vi "Error Handler.vi"(8 "Engine Error":errorcluster, 11 "Component Info In":T1) -> (0 "Engine Errors":errorcluster, 1 "Safe State":bool, 3 "Component Info Out":T1)   [LabVIEW 2013]
uses:
  Module Execution Info.ctl
  <vilib>/NI/Tag Bus Module Framework/runtime/TBM module execution interface.lvclass
  Data Table with Transfer Spec.ctl
  <vilib>/NI/Tag Bus/table/data table.ctl
  <vilib>/NI/Tag Bus/table/transfer specification.ctl
  <vilib>/NI/Tag Bus/tag/Data Type.ctl
  Configuration/Module Decimation.ctl
  Configuration/Module Error Configuration.ctl
  Configuration/Error Actions By Category.ctl
  <vilib>/NI/Tag Bus Module Framework/runtime/error classification.ctl
  Configuration/Error Actions.ctl
  error responses.ctl
  Configuration/error options.ctl
  Standard Engine Runtime.lvclass
  Configuration/Standard Engine Configuration.lvclass
  <vilib>/NI/Tag Bus/tag/tag descriptor.lvclass
  <vilib>/NI/Tag Bus/table/data table.lvlib
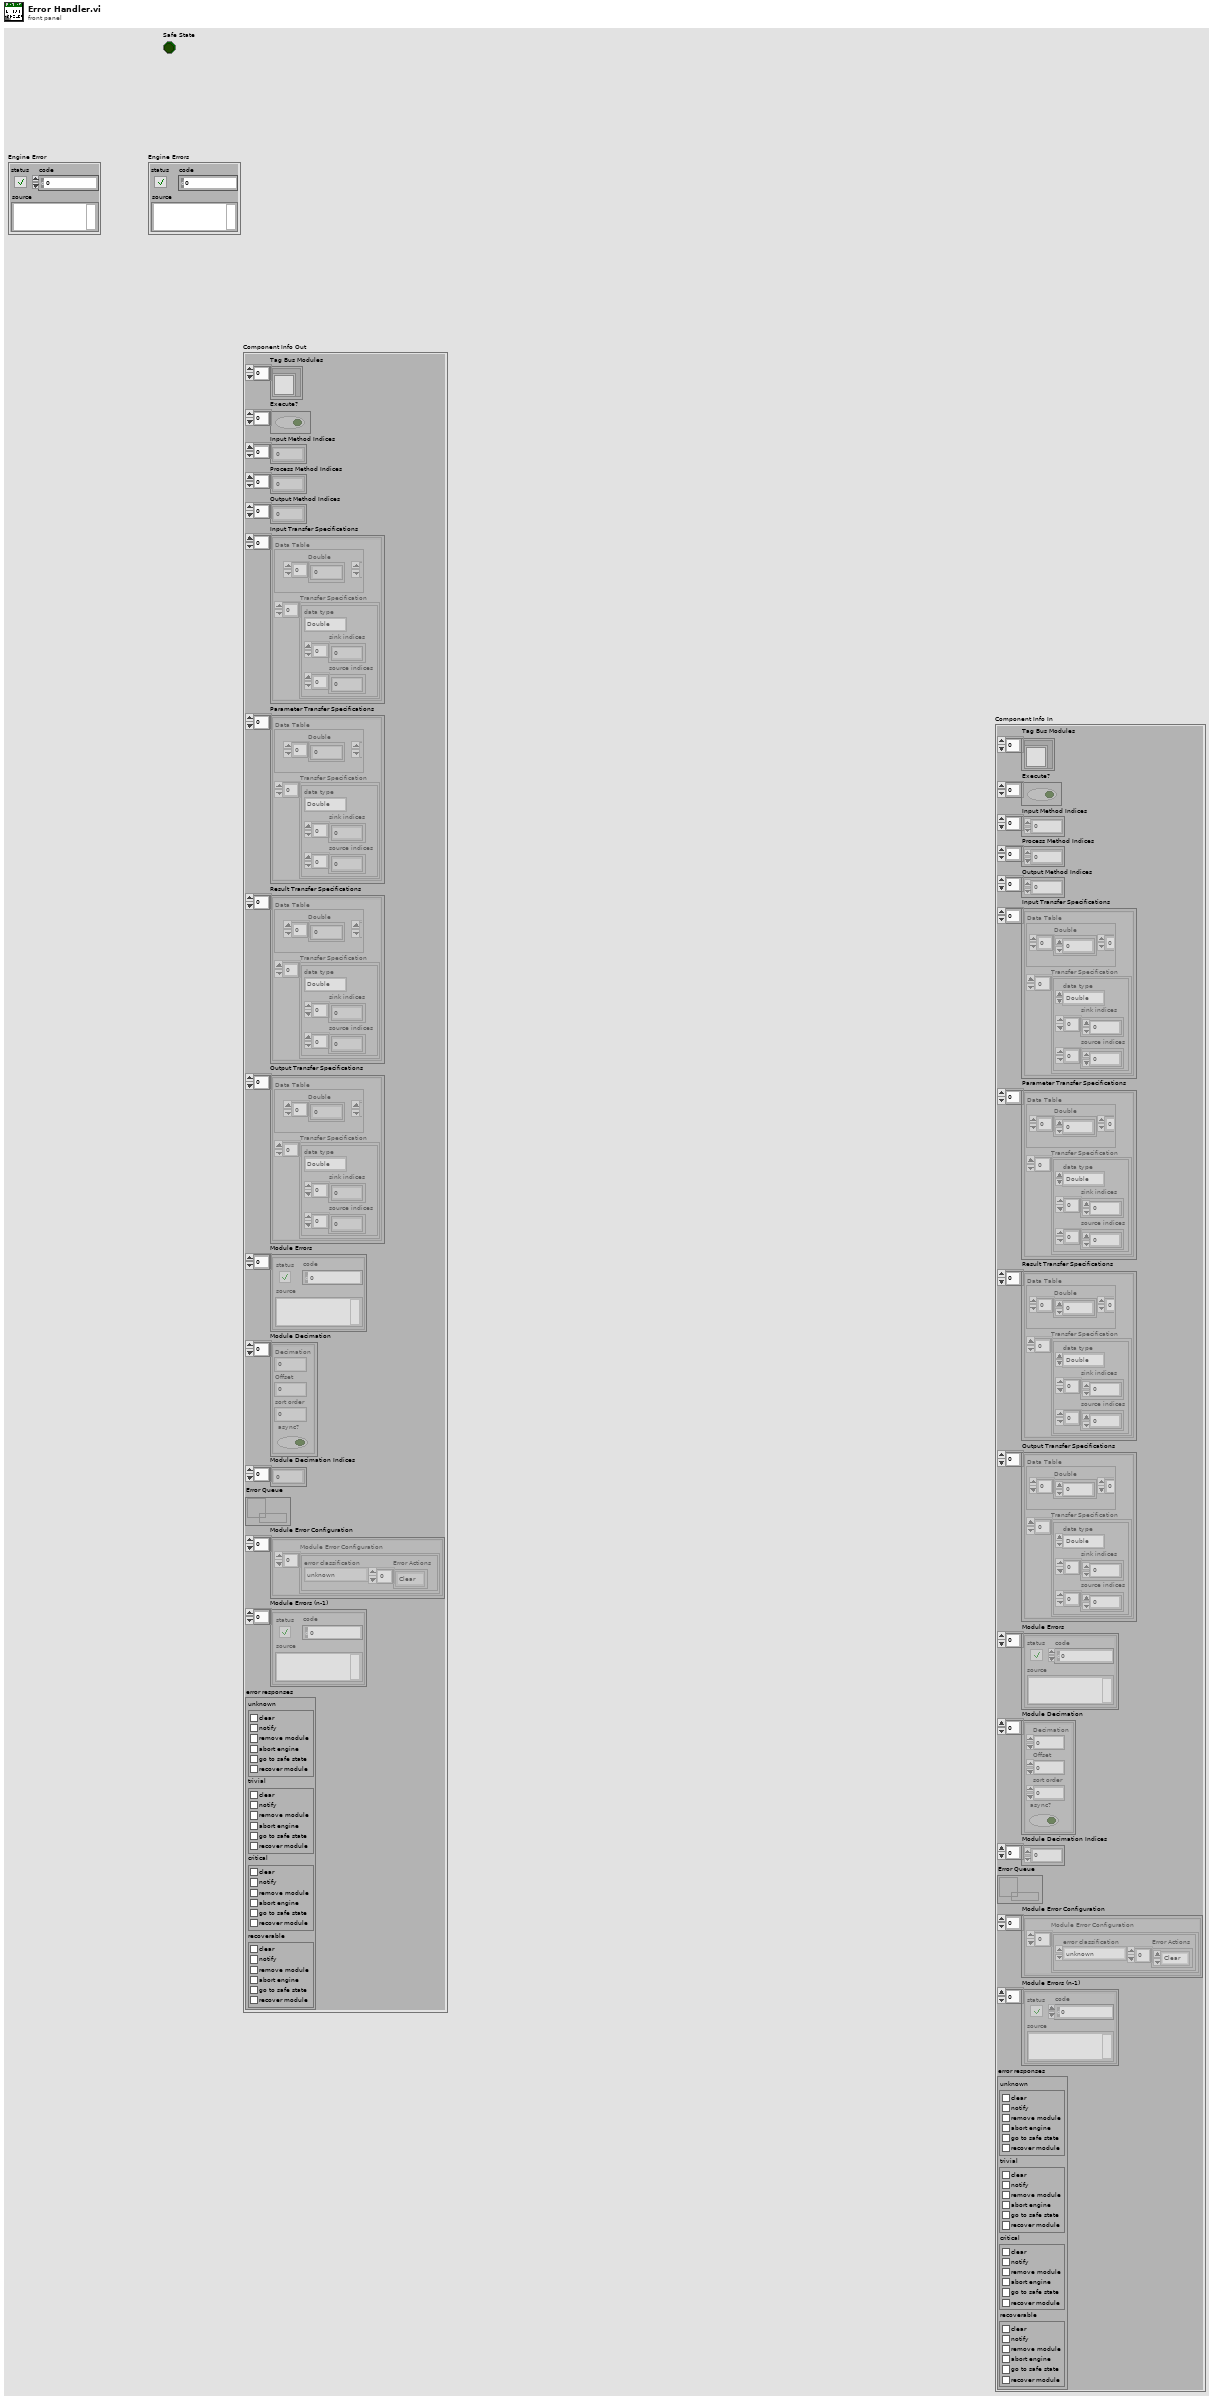
[diagram p1: front panel]
types:
  T1 = typedef "Module Execution Info.ctl" = cluster{"Tag Bus Modules":refnum<class "TBM module execution interface.lvclass">[], "Execute?":bool[], "Input Method Indices":i32[], "Process Method Indices":i32[], "Output Method Indices":i32[], "Input Transfer Specifications":T2[], "Parameter Transfer Specifications":T2[], "Result Transfer Specifications":T2[], "Output Transfer Specifications":T2[], "Module Errors":errorcluster[], "Module Decimation":T6[], "Module Decimation Indices":i32[], "Error Queue":refnum<queue>, "Module Error Configuration":T7[], "Module Errors (n-1)":errorcluster[], "error responses":T11}
  T2 = typedef "Data Table with Transfer Spec.ctl" = cluster{"Data Table":T3, "Transfer Specification":T4[]}
  T3 = typedef "tag bus.lvlib/data table.lvlib/data table.ctl" = cluster{"Double":dbl[], "Single":sgl[], "I64":i64[], "I32":i32[], "I16":i16[], "I8":i8[], "U64":u64[], "U32":u32[], "U16":u16[], "U8":u8[], "Boolean":bool[], "String":string[], "Array of Double":cluster{"DBL Array":dbl[]}[], "Array of Single":cluster{"SGL Array":sgl[]}[], "Array of I64":cluster{"I64 Array":i64[]}[], "Array of I32":cluster{"I32 Array":i32[]}[], "Array of I16":cluster{"I16 Array":i16[]}[], "Array of I8":cluster{"I8 Array":i8[]}[], "Array of U64":cluster{"U64 Array":u64[]}[], "Array of U32":cluster{"U32 Array":u32[]}[], "Array of U16":cluster{"U16 Array":u16[]}[], "Array of U8":cluster{"U8 Array":u8[]}[], "Array of Boolean":cluster{"Boolean Array":bool[]}[], "Array of String":cluster{"String Array":string[]}[]}
  T4 = typedef "tag bus.lvlib/data table.lvlib/transfer specification.ctl" = cluster{"data type":T5, "sink indices":i32[], "source indices":i32[]}
  T5 = typedef "tag bus.lvlib/tag descriptor.lvclass/Data Type.ctl" = enum16{"Double", "Single", "I64", "I32", "I16", "I8", "U64", "U32", "U16", "U8", "Boolean", "String", "Array of Double", "Array of Single", "Array of I64", "Array of I32", "Array of I16", "Array of I8", "Array of U64", "Array of U32", "Array of U16", "Array of U8", "Array of Boolean", "Array of String"}
  T6 = typedef "Standard Engine Configuration.lvclass/Module Decimation.ctl" = cluster{"Decimation":u16, "Offset":u16, "sort order":i32, "async?":bool}
  T7 = typedef "Standard Engine Configuration.lvclass/Module Error Configuration.ctl" = cluster{"Module Error Configuration":T8[]}
  T8 = typedef "Standard Engine Configuration.lvclass/Error Actions By Category.ctl" = cluster{"error classification":T9, "Error Actions":T10[]}
  T9 = typedef "TBM module execution interface.lvclass/error classification.ctl" = enum16{"unknown", "none", "trivial", "recoverable", "critical"}
  T10 = typedef "Standard Engine Configuration.lvclass/Error Actions.ctl" = enum16{"Clear", "Notify", "Stop Component", "Stop Engine", "Safe State", "Attempt Recovery"}
  T11 = typedef "Standard Engine Configuration.lvclass/error responses.ctl" = cluster{"unknown":T12, "trivial":T12, "critical":T12, "recoverable":T12}
  T12 = typedef "Standard Engine Configuration.lvclass/error options.ctl" = cluster{"clear":bool, "notify":bool, "remove module":bool, "abort engine":bool, "go to safe state":bool, "recover module":bool}
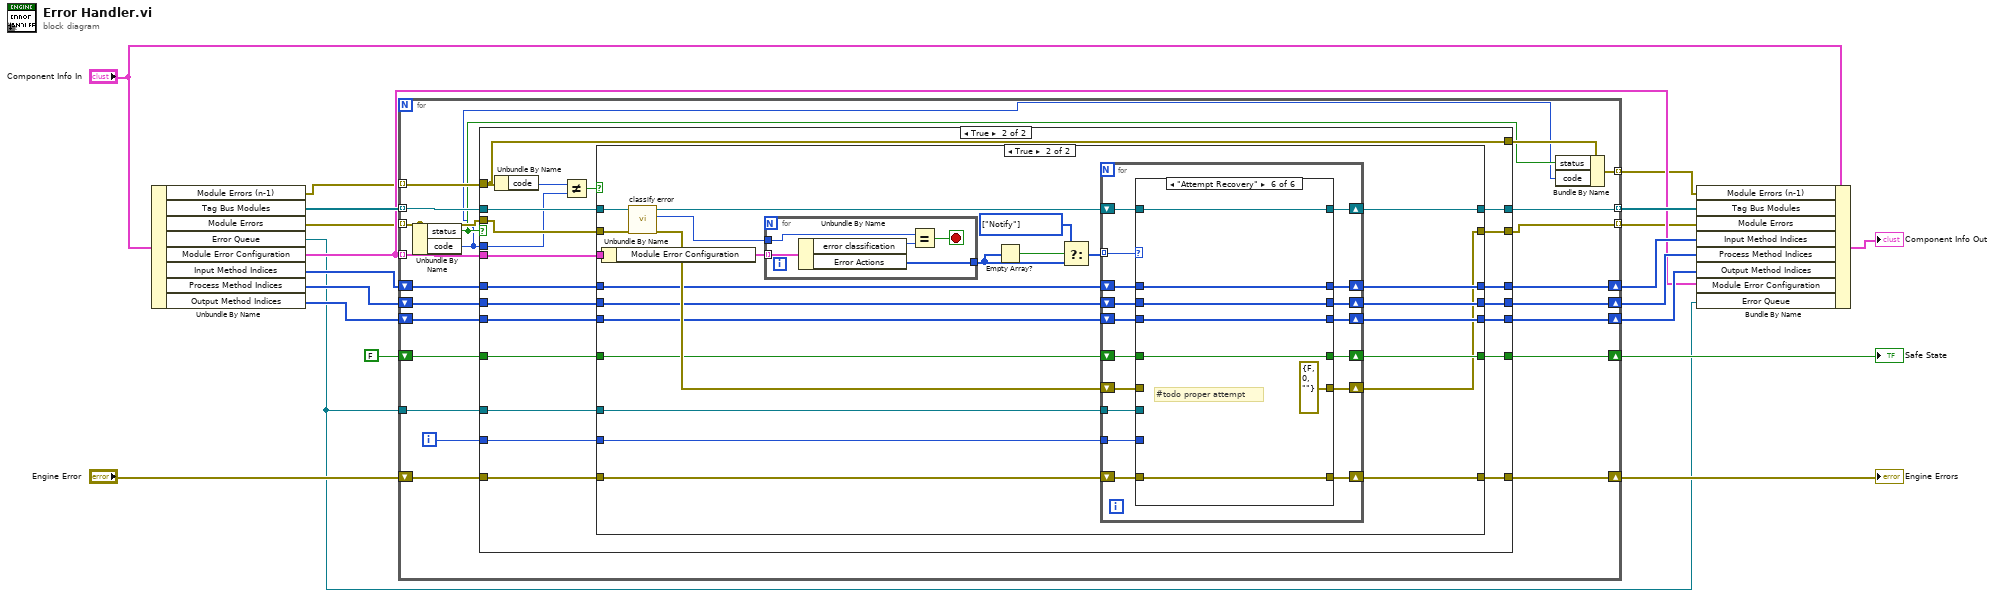
[diagram p0: block diagram]
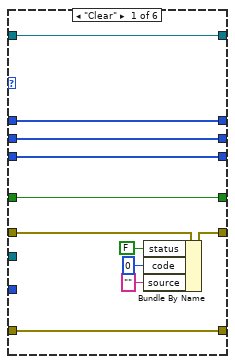
[diagram p4: hidden frame]
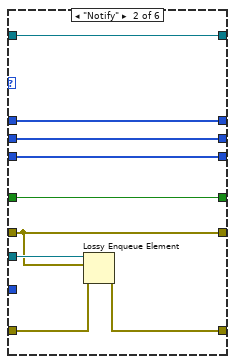
[diagram p5: hidden frame]
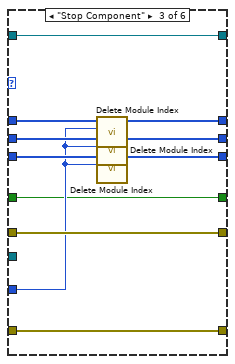
[diagram p6: hidden frame]
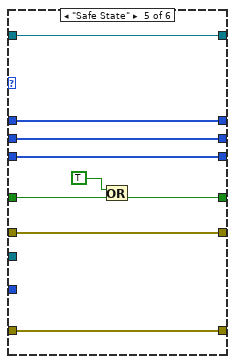
[diagram p8: hidden frame]
diagram:
  n1 = Unbundle By Name("Component Info In") -> ("Module Errors (n-1)"=w3:errorcluster[], "Tag Bus Modules"=w18:refnum<class "TBM module execution interface.lvclass">[], "Module Errors"=w4:errorcluster[], "Error Queue"=w5:refnum<queue>, "Module Error Configuration"=w6:T7[], "Input Method Indices"=w14:i32[], "Process Method Indices"=w13:i32[], "Output Method Indices"=w12:i32[])
  n2 = for {
    tunnel: w4 -> [w24] mode=indexing
    tunnel: [w40] -> w16 mode=indexing
    tunnel: w18 -> [w38] mode=indexing
    tunnel: w6 -> [w39] mode=indexing
    shift-right: [w41] -> w20
    shift-left: "Engine Error" -> [w42]
    tunnel: w5 -> [w37]
    shift-right: [w33] -> w11
    shift-left: w14 -> [w36]
    shift-right: [w32] -> w10
    shift-left: w13 -> [w35]
    shift-right: [w31] -> w9
    shift-left: w12 -> [w34]
    tunnel: w3 -> [w30] mode=indexing
    shift-right: [w29] -> w7
    shift-left: FALSE -> [w28]
    tunnel: [w26] -> w2 mode=indexing
    tunnel: [w23] -> w1 mode=indexing
    i -> [w25]
    n3 = Unbundle By Name(w24) -> ("status"=w22:bool, "code"=w21:i32)
    n4 = case shown="True" w22 {
      tunnel: w42 -> [w50 w68]
      tunnel: [w50 w67] -> w41
      tunnel: [w43 w70] -> w26
      tunnel: [w49 w69] -> w40
      tunnel: w38 -> [w49 w71]
      tunnel: w39 -> [_ w58]
      tunnel: w37 -> [_ w66]
      tunnel: w36 -> [w48 w65]
      tunnel: w35 -> [w47 w64]
      tunnel: w34 -> [w46 w63]
      tunnel: [w48 w62] -> w33
      tunnel: [w47 w61] -> w32
      tunnel: [w46 w60] -> w31
      tunnel: w25 -> [_ w59]
      tunnel: w30 -> [w44 w53]
      tunnel: [w45 w54] -> w29
      tunnel: w28 -> [w45 w55]
      tunnel: [w44 w53] -> w27
      tunnel: w24 -> [w43 w52]
      tunnel: w21 -> [_ w51]
      frame False {
      }
      frame True {
        n5 = Unbundle By Name(w53) -> ("code"=w57:i32)
        n6 = Not Equal?(x=w57, y=w51) -> (x != y?=w56:bool)
        n7 = case shown="True" w56 {
          tunnel: w71 -> [w78 w103]
          tunnel: [w77 w79] -> w70
          tunnel: [w78 w100] -> w69
          tunnel: w68 -> [w73 w99]
          tunnel: [w73 w98] -> w67
          tunnel: w66 -> [_ w97]
          tunnel: w65 -> [w76 w96]
          tunnel: w64 -> [w75 w95]
          tunnel: w63 -> [w74 w94]
          tunnel: [w76 w93] -> w62
          tunnel: [w75 w92] -> w61
          tunnel: [w74 w91] -> w60
          tunnel: w59 -> [_ w90]
          tunnel: w58 -> [_ w89]
          tunnel: w52 -> [w77 w82]
          tunnel: w55 -> [w72 w81]
          tunnel: [w72 w80] -> w54
          frame False {
          }
          frame True {
            w83 = T10[] [enum."Notify"] items=["Clear", "Notify", "Stop Component", "Stop Engine", "Safe State", "Attempt Recovery"] ("t")
            n8 = Unbundle By Name(w89) -> ("Module Error Configuration"=w88:T8[])
            n9 = call-dynamic "classify error.vi"("error to classify"=w82, "module in"=w103) -> ("classified error"=w102:errorcluster, "error classification"=w87:T9, "module out"=w101:refnum<class "TBM module execution interface.lvclass">)  [unwired: 7 in]
            n10 = for {
              tunnel: w88 -> [w178] mode=indexing
              tunnel: w87 -> [w177]
              tunnel: [w174] -> w85
              stop <- w175 stop-if-true
              n11 = Unbundle By Name(w178) -> ("error classification"=w176:T9, "Error Actions"=w174:T10[])
              n12 = Equal?(x=w177, y=w176) -> (x = y?=w175:bool)
            }
            n13 = Empty Array?(array=w85) -> (empty?=w86:bool)
            n14 = Select(t=w83, s=w86, f=w85) -> (s? t:f=w84:T10[])
            n15 = for {
              tunnel: w84 -> [w120] mode=indexing
              shift-right: [w119] -> w79
              shift-left: w102 -> [w118]
              shift-right: [w114] -> w98
              shift-left: w99 -> [w115]
              shift-right: [w117] -> w100
              shift-left: w101 -> [w116]
              tunnel: w97 -> [w113]
              shift-right: [w111] -> w93
              shift-left: w96 -> [w112]
              shift-right: [w109] -> w92
              shift-left: w95 -> [w110]
              shift-right: [w107] -> w91
              shift-left: w94 -> [w108]
              tunnel: w90 -> [w106]
              shift-right: [w104] -> w80
              shift-left: w81 -> [w105]
              n16 = case shown="\"Attempt Recovery\"" w120 {
                tunnel: [w124 w133 w151 w156 w165 errorcluster {"status"=FALSE, "code"=0, "source"=""} ("classified error")] -> w119
                tunnel: w118 -> [w125 w133 w151 w156 w165 _]
                tunnel: [w131 w140 w150 w157 w166 w173] -> w117
                tunnel: w116 -> [w131 w140 w150 w157 w166 w173]
                tunnel: w115 -> [w130 w134 w149 _ w161 w172]
                tunnel: [w130 w138 w149 w156 w161 w172] -> w114
                tunnel: w113 -> [_ w139 _ _ _ _]
                tunnel: w112 -> [w129 w137 w148 w155 w164 w171]
                tunnel: [w129 w137 w147 w155 w164 w171] -> w111
                tunnel: w110 -> [w128 w136 w146 w154 w163 w170]
                tunnel: [w128 w136 w144 w154 w163 w170] -> w109
                tunnel: w108 -> [w127 w135 w145 w153 w162 w169]
                tunnel: [w127 w135 w143 w153 w162 w169] -> w107
                tunnel: w106 -> [_ _ w142 _ _ _]
                tunnel: w105 -> [w126 w132 w141 w152 w160 w168]
                tunnel: [w126 w132 w141 w152 w159 w168] -> w104
                frame "Clear" {
                  n17 = Bundle By Name(cluster=w125, "status"=FALSE, "code"=0, "source"="") -> (w124:errorcluster)
                }
                frame "Notify" {
                  n18 = Lossy Enqueue Element(queue=w139, element=w133, error in (no error)=w134) -> (error out=w138:errorcluster)  [unwired: 3 out]
                }
                frame "Stop Component" {
                  n19 = call "Delete Module Index.vi"("Index"=w142, "Module Indices"=w148) -> ("Module Indices"=w147:i32[])  [unwired: 9 in]
                  n20 = call "Delete Module Index.vi"("Index"=w142, "Module Indices"=w146) -> ("Module Indices"=w144:i32[])  [unwired: 9 in]
                  n21 = call "Delete Module Index.vi"("Index"=w142, "Module Indices"=w145) -> ("Module Indices"=w143:i32[])  [unwired: 9 in]
                }
                frame "Stop Engine" {
                  # "Passing an engine error out stops the engine."
                }
                frame "Safe State" {
                  n22 = Or(x=TRUE ("Stop Engine"), y=w160) -> (x .or. y?=w159:bool)
                }
                frame "Attempt Recovery" {
                  # "#todo proper attempt"
                }
              }
            }
          }
        }
      }
    }
    n23 = Bundle By Name(cluster=w27, "status"=w22, "code"=w21) -> (w23:errorcluster)
  }
  "Engine Errors" <- w20
  "Safe State" <- w7
  n24 = Bundle By Name(cluster="Component Info In", "Module Errors (n-1)"=w1, "Tag Bus Modules"=w16, "Module Errors"=w2, "Input Method Indices"=w11, "Process Method Indices"=w10, "Output Method Indices"=w9, "Module Error Configuration"=w6, "Error Queue"=w5) -> (→"Component Info Out":T1)
